vi "AuMT8852B Signal Generator Configuration.vi"(5 "Settings":T1={"Pattern"=enum."CW", "RF state"=enum."RF on", "TX/RX frequency"=0.0, "Modulation index"=0.25, "Power (dBm)"=0.0, "Frequency units"=enum."MHz"} {"Power (dBm)" format="%.2f"; "Modulation index" format="%.2f"; "TX/RX frequency" format="%.2f"}, 7 "Set/Get (Set)":enum16{"Set", "Get"}(ring), 8 "error in (no error)":errorcluster, 11 "VISA session":refnum<visa-resource-name>) -> (0 "error out":errorcluster, 2 "error code":i32, 3 "VISA session out":refnum<visa-resource-name>, 4 "Settings out":T1={"Pattern"=enum."CW", "RF state"=enum."RF on", "TX/RX frequency"=0.0, "Modulation index"=0.25, "Power (dBm)"=0.0, "Frequency units"=enum."MHz"} {"Power (dBm)" format="%.2f"; "Modulation index" format="%.2f"; "TX/RX frequency" format="%.2f"})   [LabVIEW 2017]
doc: "Anritsu MT8852B Bluetooth Tester\n\nConfigures the Signal Generator mode. To enter Signal Generator mode, use the Operation Mode command.\n\nINPUTS\nSet/Get - whether to send or retrieve the parameters.\nSettings - new parameters of the signal generator mode.\n\nOUTPUTS\nSettings out - current parameters of the signal generator mode."
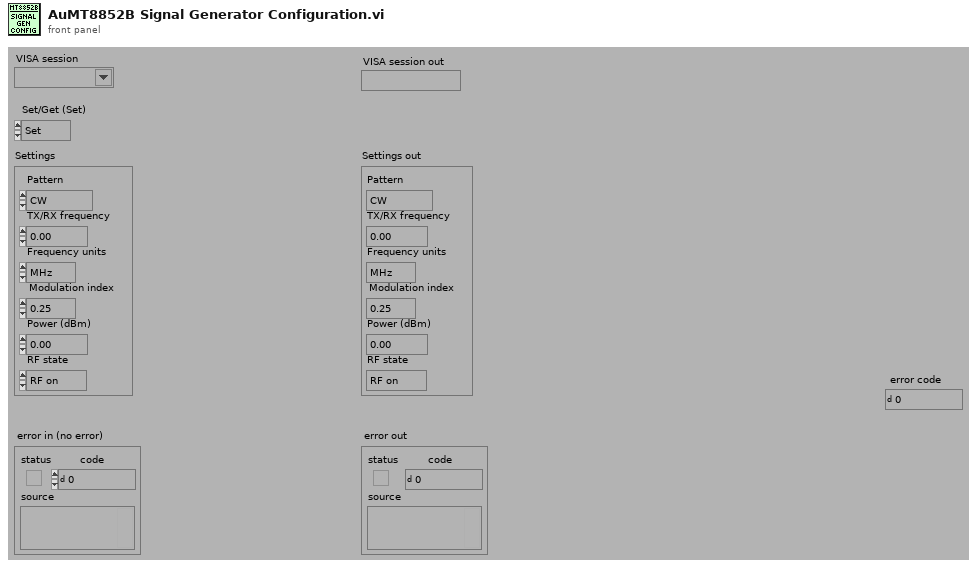
[diagram p1: front panel]
types:
  T1 = cluster{"Pattern":enum16{"CW", "10101010", "11110000", "PRBS9", "PRBS15"}, "RF state":enum16{"RF off", "RF on"}, "TX/RX frequency":dbl, "Modulation index":dbl, "Power (dBm)":dbl, "Frequency units":enum16{"Channel", "MHz"}}
  T2 = enum16{"Simulate", "Range check", "Cache", "Query instrument status"}
  T3 = enum16{"CW", "10101010", "11110000", "PRBS9", "PRBS15"}
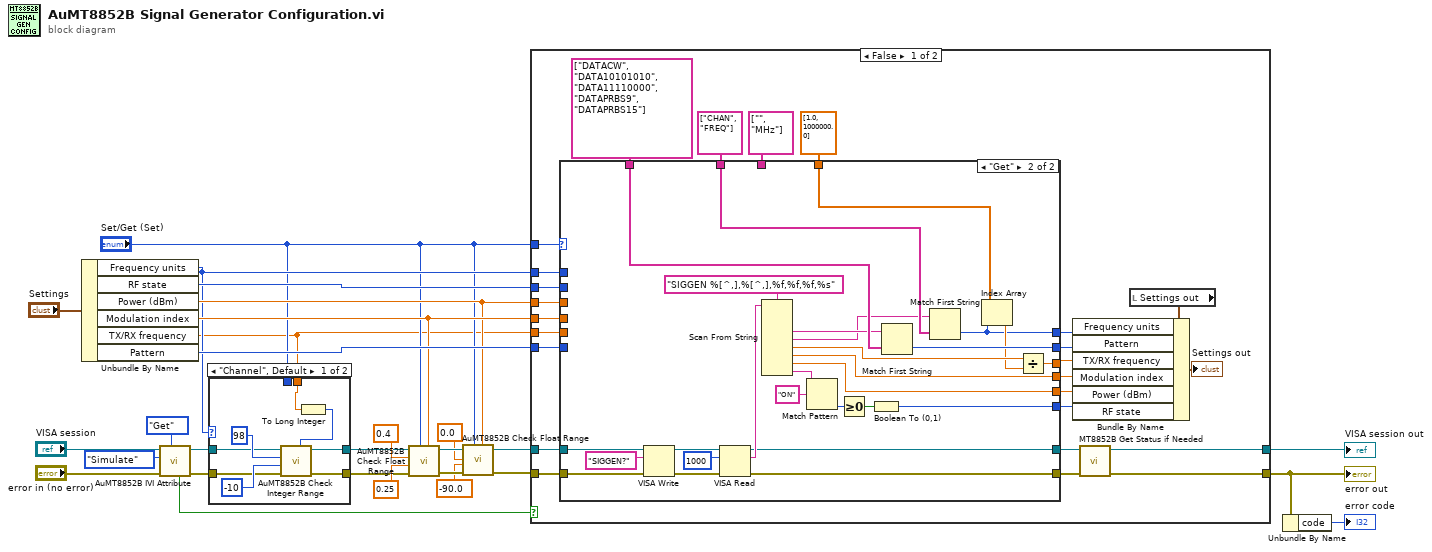
[diagram p0: block diagram]
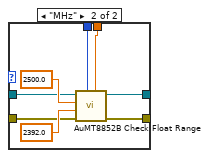
[diagram p2: hidden frame]
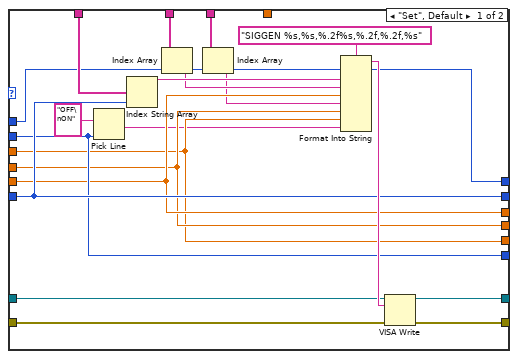
[diagram p3: hidden frame]
diagram:
  n1 = Unbundle By Name("Settings") -> ("Frequency units"=w3:enum16{"Channel", "MHz"}, "RF state"=w8:enum16{"RF off", "RF on"}, "Power (dBm)"=w9:dbl, "Modulation index"=w10:dbl, "TX/RX frequency"=w1:dbl, "Pattern"=w11:T3)
  n2 = call <instrlib>:"AuMT8852B IVI Attribute.vi"("Set/Get (Set)"=enum16{"Set", "Get"}."Get", "error in (no error)"="error in (no error)", "Flag (Simulate)"=T2."Simulate", "VISA session"="VISA session") -> ("error out"=w7:errorcluster, "VISA session out"=w6:refnum<visa-resource-name>, "Value out"=w23:bool)  [unwired: 5 in]
  n3 = case shown="\"Channel\", Default" w3 {
    tunnel: [w34 w44] -> w5
    tunnel: [w33 w43] -> w4
    tunnel: w7 -> [w30 w40]
    tunnel: w6 -> [w29 w39]
    tunnel: "Set/Get (Set)" -> [_ w38]
    tunnel: w1 -> [w31 w37]
    frame "Channel", Default {
      n4 = To Long Integer(number=w31) -> (32bit integer=w32:i32)
      n5 = call <instrlib>:"AuMT8852B Check Integer Range.vi"("Value (0)"=w32, "error in (no error)"=w30, "Lower limit (-1)"=-10, "Upper limit (1)"=98, "VISA session"=w29) -> ("error out"=w34:errorcluster, "VISA session out"=w33:refnum<visa-resource-name>)  [unwired: 5 in]
    }
    frame "MHz" {
      n6 = call <instrlib>:"AuMT8852B Check Float Range.vi"("Value (0)"=w37, "Set/Get (Set)"=w38, "error in (no error)"=w40, "Lower limit (-1)"=2392.0, "Upper limit (1)"=2500.0, "VISA session"=w39) -> ("error out"=w44:errorcluster, "VISA session out"=w43:refnum<visa-resource-name>)  [unwired: 4 in]
    }
  }
  n7 = call <instrlib>:"AuMT8852B Check Float Range.vi"("Value (0)"=w10, "Set/Get (Set)"="Set/Get (Set)", "error in (no error)"=w5, "Lower limit (-1)"=0.25, "Upper limit (1)"=0.4, "VISA session"=w4) -> ("error out"=w17:errorcluster, "VISA session out"=w16:refnum<visa-resource-name>)  [unwired: 4 in]
  n8 = call <instrlib>:"AuMT8852B Check Float Range.vi"("Value (0)"=w9, "Set/Get (Set)"="Set/Get (Set)", "error in (no error)"=w17, "Lower limit (-1)"=-90.0, "Upper limit (1)"=0.0, "VISA session"=w16) -> ("error out"=w13:errorcluster, "VISA session out"=w12:refnum<visa-resource-name>)  [unwired: 4 in]
  n9 = case shown="False" w23 {
    tunnel: [w51 w118] -> w28
    tunnel: [w52 w117] -> w21
    tunnel: w13 -> [w64 w117]
    tunnel: w12 -> [w63 w118]
    tunnel: w11 -> [w69 _]
    tunnel: w1 -> [w68 _]
    tunnel: w10 -> [w67 _]
    tunnel: w9 -> [w66 _]
    tunnel: w8 -> [w65 _]
    tunnel: "Set/Get (Set)" -> [w62 _]
    tunnel: w3 -> [w48 _]
    frame False {
      n10 = case shown="\"Get\"" w62 {
        tunnel: [w80 w98] -> w54
        tunnel: [w79 w97] -> w53
        tunnel: w69 -> [w82 _]
        tunnel: w68 -> [w76 _]
        tunnel: w67 -> [w72 _]
        tunnel: w66 -> [w71 _]
        tunnel: w65 -> [w81 _]
        tunnel: w64 -> [w85 w115]
        tunnel: w63 -> [w84 w114]
        tunnel: string[] ["DATACW", "DATA10101010", "DATA11110000", "DATAPRBS9", "DATAPRBS15"] ("Array Constant") -> [w83 w109]
        tunnel: [w72 w107] -> w57
        tunnel: [w71 w106] -> w56
        tunnel: [w81 w101] -> w55
        tunnel: [w82 w100] -> w60
        tunnel: [w76 w94] -> w58
        tunnel: string[] ["CHAN", "FREQ"] ("Array Constant") -> [w78 w96]
        tunnel: string[] ["", "MHz"] ("Array Constant") -> [w75 _]
        tunnel: w48 -> [w74 _]
        tunnel: [w74 w90] -> w47
        tunnel: dbl[] [1.0, 1000000.0] ("Array Constant") -> [_ w92]
        frame "Set", Default {
          n11 = Pick Line(multi-line string="OFF\nON", line index=w81) -> (output string=w70:string)  [unwired: 1 in]
          n12 = Index String Array(1:w82, 2:w83) -> (0:w87:string)  [unwired: 1 in]
          n13 = Index Array(array=w78, index=w74) -> (element=w77:string)
          n14 = Index Array(array=w75, index=w74) -> (element=w73:string)
          n15 = Format Into String(format string="SIGGEN %s,%s,%.2f%s,%.2f,%.2f,%s" ("Format String"), w87, w77, w76, w73, w72, w71, w70) -> (resulting string=w86:string)  [unwired: 2 in, 1 out]
          n16 = VISA Write(VISA resource name=w84, write buffer=w86, error in (no error)=w85) -> (VISA resource name out=w80:refnum<visa-resource-name>, error out=w79:errorcluster)  [unwired: 1 out]
        }
        frame "Get" {
          n17 = VISA Write(VISA resource name=w114, write buffer="SIGGEN?" ("write buffer (\"\")"), error in (no error)=w115) -> (VISA resource name out=w111:refnum<visa-resource-name>, error out=w112:errorcluster)  [unwired: 1 out]
          n18 = VISA Read(VISA resource name=w111, byte count=u32 1000 ("byte count (0)"), error in (no error)=w112) -> (VISA resource name out=w98:refnum<visa-resource-name>, read buffer=w99:string, error out=w97:errorcluster)  [unwired: 1 out]
          n19 = Scan From String(format string="SIGGEN %[^,],%[^,],%f,%f,%f,%s" ("Format String"), input string=w99) -> (output 1=w108:string, output 2=w95:string, output 3=w93:dbl, output 4=w107:dbl, output 5=w106:dbl, output 6=w104:string)  [unwired: 8 in, 3 out]
          n20 = Match Pattern(string=w104, regular expression="ON") -> (offset past match=w103:i32)  [unwired: 1 in, 3 out]
          n21 = Greater Or Equal To 0?(x=w103) -> (x >= 0?=w102:bool)
          n22 = Boolean To (0,1)(Boolean=w102) -> (0, 1=w101:i16)
          n23 = Match First String(2:w109, 3:w108) -> (0:w100:i32)  [unwired: 1 out]
          n24 = Match First String(2:w96, 3:w95) -> (0:w90:i32)  [unwired: 1 out]
          n25 = Index Array(array=w92, index=w90) -> (element=w91:dbl)
          n26 = Divide(x=w93, y=w91) -> (x/y=w94:dbl)
        }
      }
      n27 = call <instrlib>:"MT8852B Get Status if Needed.vi"("error in (no error)"=w53, "VISA session"=w54) -> ("error out"=w52:errorcluster, "VISA session out"=w51:refnum<visa-resource-name>)  [unwired: 8 in]
      n28 = local read "Settings out"() -> (w59:T1)
      n29 = Bundle By Name(cluster=w59, "Frequency units"=w47, "Pattern"=w60, "TX/RX frequency"=w58, "Modulation index"=w57, "Power (dBm)"=w56, "RF state"=w55) -> (→"Settings out":T1)
    }
    frame True {
    }
  }
  "error out" <- w21
  "VISA session out" <- w28
  n30 = Unbundle By Name(w21) -> ("code"=→"error code":i32)
